vi "CheckImagePoly.vi"   [LabVIEW 2015]
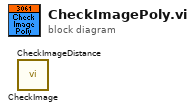
[diagram p0: block diagram]
diagram:
  n1 = call "CheckImage.vi"() -> ()  [unwired: 9 in, 3 out]
  n2 = call "CheckImageDistance.vi"() -> ()  [unwired: 8 in, 4 out]
